vi "lecroy_enable.vi"(0 "VISA in":refnum<visa-resource-name>, 1 "Enable":bool, 2 "Crate":i32, 3 "Card":dbl, 4 "Channel":dbl, 5 "error in":errorcluster, 7 "Num Channels":i32=1) -> (14 "VISA out":refnum<visa-resource-name>, 16 "Read Channel Voltage":dbl, 19 "error out":errorcluster)   [LabVIEW 2018]
uses:
  General_lecroy_command.ctl
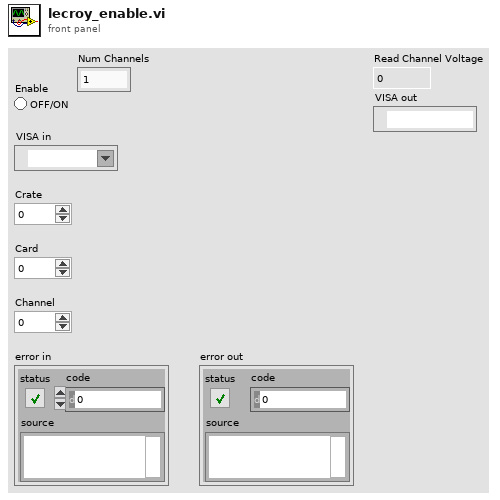
[diagram p1: front panel]
types:
  T1 = enum16{"Monitor", "Demand", "Backup", "All", "None"}
  T2 = typedef "General_lecroy_command.ctl" = string
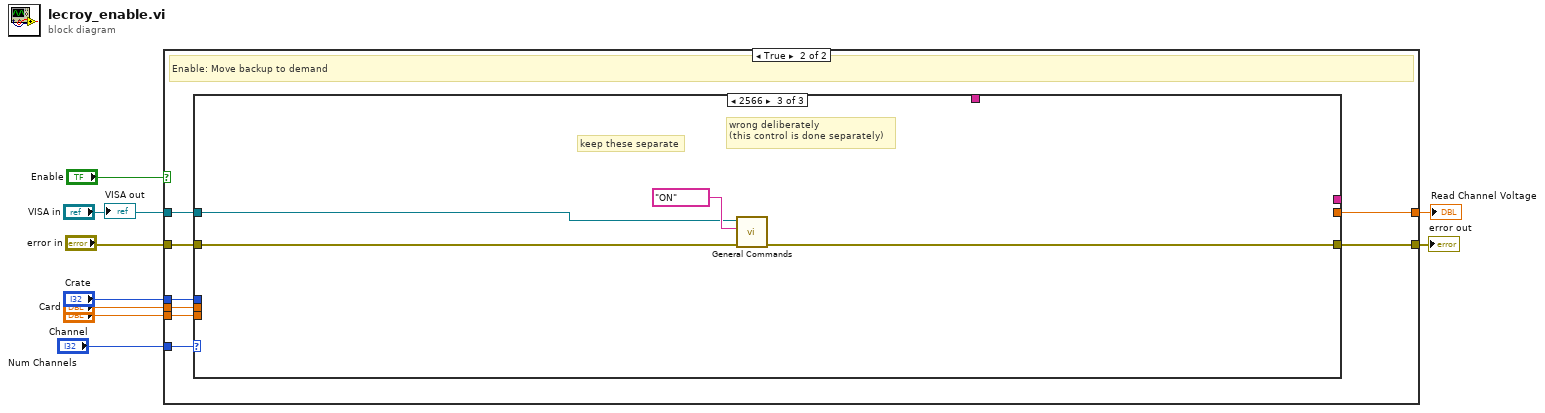
[diagram p0: block diagram]
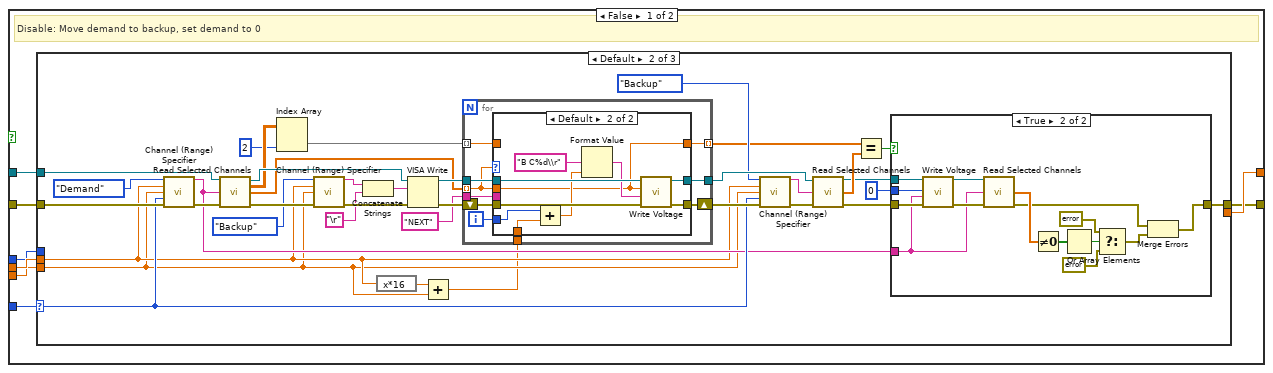
[diagram p2: hidden frame]
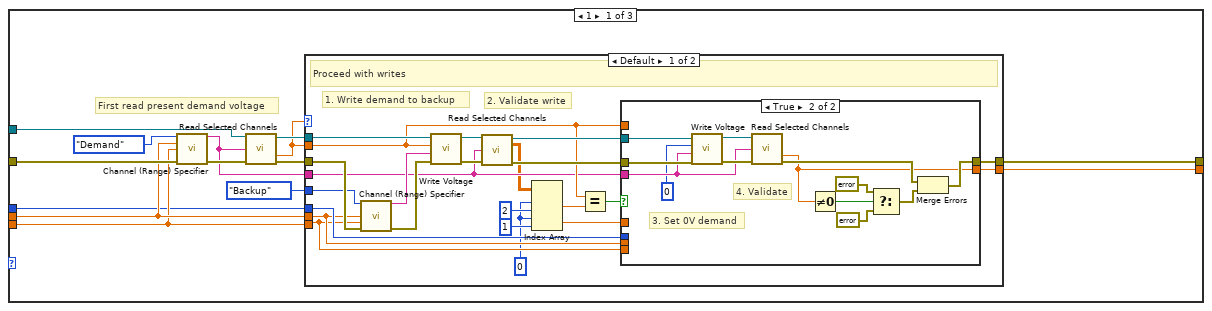
[diagram p3: hidden frame]
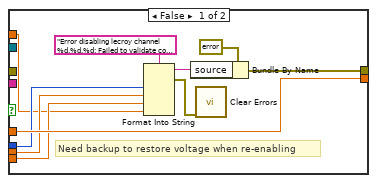
[diagram p4: hidden frame]
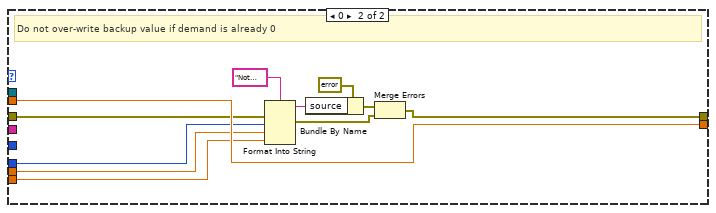
[diagram p5: hidden frame]
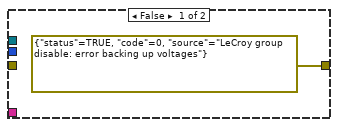
[diagram p6: hidden frame]
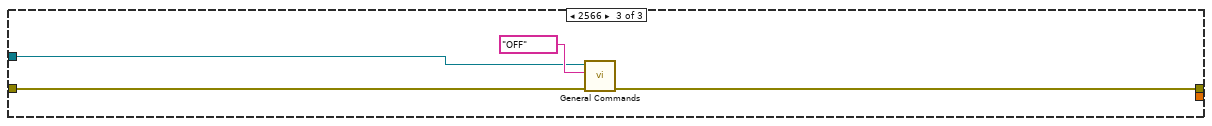
[diagram p8: hidden frame]
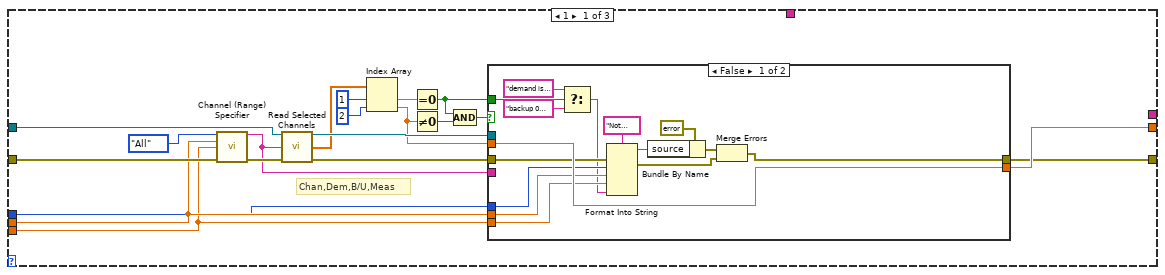
[diagram p9: hidden frame]
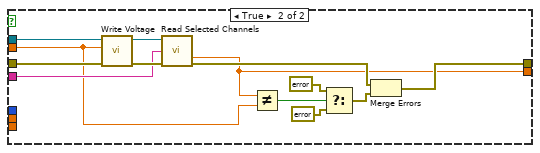
[diagram p10: hidden frame]
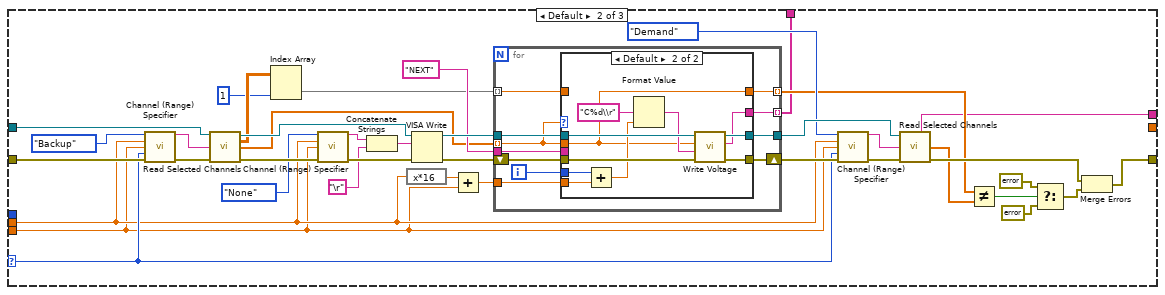
[diagram p11: hidden frame]
diagram:
  n1 = case shown="True" "Enable" {
    tunnel: [w11 w168] -> w2
    tunnel: [w12 w169] -> w3
    tunnel: "error in" -> [w16 w173]
    tunnel: "Channel" -> [w14 w171]
    tunnel: "Card" -> [w15 w172]
    tunnel: "VISA in" -> [w17 w174]
    tunnel: "Crate" -> [w13 w170]
    tunnel: "Num Channels" -> [w10 w167]
    frame False {
      # "Disable: Move demand to backup, set demand to 0"
      n2 = case shown="Default" w10 {
        selector: w10 -> [_ w104 _]
        tunnel: w17 -> [w30 w106 w165]
        tunnel: w16 -> [w29 w105 w164]
        tunnel: w15 -> [w25 w91 _]
        tunnel: w14 -> [w24 w90 _]
        tunnel: w13 -> [w23 _ _]
        tunnel: [w22 _ _] -> w12
        tunnel: [w21 w103 w163] -> w11
        frame 1 {
          # "First read present demand voltage"
          n3 = call "Channel (Range) Specifier.vi"("Buffer"=T1."Demand", "Card"=w25, "Channel"=w24, "error in"=w29) -> ("Channel (Range)"=w26:string, "error out"=w31:errorcluster)  [unwired: 10 in]
          n4 = call "Read Selected Channels.vi"("VISA in"=w30, "C##,##DO###"=w26, "error in"=w31) -> ("VISA out"=w28:refnum<visa-resource-name>, "First Value"=w18:dbl, "error out"=w27:errorcluster)  [unwired: 6 in, 4 out]
          n5 = case shown="Default" w18 {
            tunnel: [w54 w84] -> w22
            tunnel: [w53 w86] -> w21
            tunnel: w18 -> [w38 w84]
            tunnel: w28 -> [w52 _]
            tunnel: w27 -> [w51 w79]
            tunnel: w26 -> [w36 _]
            tunnel: w25 -> [w40 w81]
            tunnel: w24 -> [w39 w82]
            tunnel: w23 -> [w41 w80]
            tunnel: T1."Backup" ("Buffer") -> [w42 _]
            frame Default {
              w32 = 0 ("disabled index (col)")
              # "2. Validate write"
              # "1. Write demand to backup"
              # "Proceed with writes"
              n6 = call "Channel (Range) Specifier.vi"("Buffer"=w42, "Channel"=w40, "Num Channels"=w39, "error in"=w51) -> ("Channel (Range)"=w37:string, "error out"=w50:errorcluster)  [unwired: 10 in]
              n7 = call "Write Voltage.vi"("error in"=w50, "Channel+Range"=w37, "Voltage input"=w38, "VISA in"=w52) -> ("error out"=w49:errorcluster, "VISA out"=w48:refnum<visa-resource-name>)  [unwired: 5 in, 1 out]
              n8 = call "Read Selected Channels.vi"("VISA in"=w48, "C##,##DO###"=w36, "error in"=w49) -> ("VISA out"=w46:refnum<visa-resource-name>, "Channel Array"=w35:dbl[][], "error out"=w47:errorcluster)  [unwired: 6 in, 4 out]
              n9 = Index Array(array=w35, index (row) #1=w32, index (col) #1=2 ("disabled index (col)"), index (row) #2=w32, index (col) #2=1 ("disabled index (col)")) -> (element #1=w44:dbl, element #2=w43:dbl)
              n10 = Equal?(x=w38, y=w44) -> (x = y?=w45:bool)
              n11 = case shown="True" w45 {
                tunnel: [w64 w65] -> w54
                tunnel: [w61 w66] -> w53
                tunnel: w36 -> [_ w73]
                tunnel: w47 -> [_ w77]
                tunnel: w46 -> [_ w76]
                tunnel: w43 -> [w64 _]
                tunnel: w41 -> [w59 _]
                tunnel: w40 -> [w58 _]
                tunnel: w39 -> [w57 _]
                tunnel: w38 -> [w56 _]
                frame False {
                  # "Need backup to restore voltage when re-enabling"
                  n12 = Format Into String(format string="Error disabling lecroy channel %d.%d.%d: Failed to validate copy of demand voltage %d to backup" ("source"), w59, w58, w57, w56) -> (resulting string=w62:string, error out=w55:errorcluster)  [unwired: 2 in]
                  n13 = Bundle By Name(cluster=errorcluster {"status"=TRUE, "code"=0, "source"=""} ("error out"), "source"=w62) -> (w61:errorcluster)
                  n14 = call <vilib>:"Clear Errors.vi"("error in (no error)"=w55) -> ()  [unwired: 5 in, 2 out]
                }
                frame True {
                  # "3. Set 0V demand"
                  # "4. Validate"
                  n15 = call "Write Voltage.vi"("error in"=w77, "Channel+Range"=w73, "Voltage input"=0, "VISA in"=w76) -> ("error out"=w75:errorcluster, "VISA out"=w74:refnum<visa-resource-name>)  [unwired: 5 in, 1 out]
                  n16 = call "Read Selected Channels.vi"("VISA in"=w74, "C##,##DO###"=w73, "error in"=w75) -> ("First Value"=w65:dbl, "error out"=w67:errorcluster)  [unwired: 6 in, 5 out]
                  n17 = Not Equal To 0?(x=w65) -> (x != 0?=w69:bool)
                  n18 = Select(t=errorcluster {"status"=TRUE, "code"=0, "source"="LeCroy disable validation error"} ("error out"), s=w69, f=errorcluster {"status"=FALSE, "code"=0, "source"=""} ("error out")) -> (s? t:f=w68:errorcluster)
                  n19 = Merge Errors(w67, w68) -> (w66:errorcluster)
                }
              }
            }
            frame 0 {
              # "Do not over-write backup value if demand is already 0"
              n20 = Format Into String(format string="Not enabling channel %d.%d.%d:\ndemand is 0 (channel already disabled)" ("source"), error in=w79, w80, w81, w82) -> (resulting string=w87:string, error out=w83:errorcluster)  [unwired: 1 in]
              n21 = Bundle By Name(cluster=errorcluster {"status"=TRUE, "code"=0, "source"=""} ("error out"), "source"=w87) -> (w85:errorcluster)
              n22 = Merge Errors(w85, w83) -> (w86:errorcluster)
            }
          }
        }
        frame Default {
          n23 = call "Channel (Range) Specifier.vi"("Buffer"=T1."Demand", "Card"=w91, "Channel"=w90, "Num Channels"=w104, "error in"=w105) -> ("Channel (Range)"=w93:string, "error out"=w124:errorcluster)  [unwired: 9 in]
          n24 = call "Read Selected Channels.vi"("VISA in"=w106, "C##,##DO###"=w93, "error in"=w124) -> ("VISA out"=w120:refnum<visa-resource-name>, "Channel Array"=w98:dbl[][], "Selected Buffer"=w101:dbl[], "error out"=w122:errorcluster)  [unwired: 6 in, 3 out]
          n25 = Index Array(array=w98, index (col)=2 ("disabled index (col)")) -> (element=w96:dbl[])  [unwired: 1 in]
          n26 = call "Channel (Range) Specifier.vi"("Buffer"=T1."Backup", "Card"=w91, "Channel"=w90, "error in"=w122) -> ("Channel (Range)"=w118:string, "error out"=w116:errorcluster)  [unwired: 10 in]
          n27 = Concatenate Strings(w118, "\r") -> (w117:string)
          n28 = expression code="x*16"(w91) -> (w92:dbl)
          n29 = VISA Write(VISA resource name=w120, write buffer=w117, error in (no error)=w116) -> (VISA resource name out=w119:refnum<visa-resource-name>, error out=w121:errorcluster)  [unwired: 1 out]
          n30 = Add(x=w92, y=w90) -> (x+y=w89:dbl)
          n31 = for {
            shift-right: [w149] -> w115
            shift-left: w121 -> [w147]
            tunnel: w119 -> [w146]
            tunnel: [w148] -> w113
            tunnel: w101 -> [w143] mode=indexing
            tunnel: "NEXT" ("Channel (Range)") -> [w145]
            tunnel: [w144] -> w99 mode=indexing
            tunnel: w96 -> [w142] mode=indexing
            tunnel: w89 -> [w140]
            i -> [w141]
            n32 = case shown="Default" w143 {
              tunnel: [w151 w162] -> w149
              tunnel: [w150 w161] -> w148
              tunnel: w147 -> [w151 w160]
              tunnel: w146 -> [w150 w159]
              tunnel: w143 -> [_ w153]
              tunnel: w145 -> [_ _]
              tunnel: [w152 w153] -> w144
              tunnel: w142 -> [w152 _]
              tunnel: w141 -> [_ w158]
              tunnel: w140 -> [_ w157]
              frame 0 {
              }
              frame Default {
                n33 = Add(x=w158, y=w157) -> (x+y=w155:dbl)
                n34 = Format Value(format string="B C%d\\r" ("Channel (Range)"), value (0)=w155) -> (output string=w154:string)  [unwired: 1 in]
                n35 = call "Write Voltage.vi"("error in"=w160, "Channel+Range"=w154, "Voltage input"=w153, "VISA in"=w159) -> ("error out"=w162:errorcluster, "VISA out"=w161:refnum<visa-resource-name>)  [unwired: 5 in, 1 out]
              }
            }
          }
          n36 = call "Channel (Range) Specifier.vi"("Buffer"=T1."Backup", "Card"=w91, "Channel"=w90, "Num Channels"=w104, "error in"=w115) -> ("Channel (Range)"=w112:string, "error out"=w114:errorcluster)  [unwired: 9 in]
          n37 = call "Read Selected Channels.vi"("VISA in"=w113, "C##,##DO###"=w112, "error in"=w114) -> ("VISA out"=w95:refnum<visa-resource-name>, "Selected Buffer"=w102:dbl[], "error out"=w123:errorcluster)  [unwired: 6 in, 4 out]
          n38 = Equal?(x=w99, y=w102) -> (x = y?=w100:bool)
          n39 = case shown="True" w100 {
            tunnel: w123 -> [_ w133]
            tunnel: [errorcluster {"status"=TRUE, "code"=0, "source"="LeCroy group disable: error backing up voltages"} ("error out") w136] -> w103
            tunnel: w95 -> [_ w132]
            tunnel: 0 ("Voltage input") -> [_ w131]
            tunnel: w93 -> [_ w128]
            frame False {
            }
            frame True {
              n40 = call "Write Voltage.vi"("error in"=w133, "Channel+Range"=w128, "Voltage input"=w131, "VISA in"=w132) -> ("error out"=w130:errorcluster, "VISA out"=w129:refnum<visa-resource-name>)  [unwired: 5 in, 1 out]
              n41 = call "Read Selected Channels.vi"("VISA in"=w129, "C##,##DO###"=w128, "error in"=w130) -> ("Selected Buffer"=w127:dbl[], "error out"=w126:errorcluster)  [unwired: 6 in, 5 out]
              n42 = Not Equal To 0?(x=w127) -> (x != 0?=w135:bool[])
              n43 = Or Array Elements(Boolean array=w135) -> (logical OR=w134:bool)
              n44 = Select(t=errorcluster {"status"=TRUE, "code"=0, "source"="LeCroy group enable validation error"} ("error out"), s=w134, f=errorcluster {"status"=FALSE, "code"=0, "source"=""} ("error out")) -> (s? t:f=w139:errorcluster)
              n45 = Merge Errors(w126, w139) -> (w136:errorcluster)
            }
          }
        }
        frame 2566 {
          n46 = call "General Commands.vi"("error in"=w164, "Action"=T2 "OFF", "VISA in"=w165) -> ("error out"=w163:errorcluster)  [unwired: 6 in, 2 out]
        }
      }
    }
    frame True {
      # "Enable: Move backup to demand"
      n47 = case shown="2566" w167 {
        selector: w167 -> [_ w234 _]
        tunnel: w174 -> [w193 w260 w288]
        tunnel: w173 -> [w192 w259 w287]
        tunnel: w172 -> [w184 w227 _]
        tunnel: w171 -> [w183 w226 _]
        tunnel: w170 -> [w182 _ _]
        tunnel: [w181 _ _] -> w169
        tunnel: [w180 w257 w289] -> w168
        tunnel: [_ w225 _] -> _
        tunnel: [_ w223 _] -> _
        frame 1 {
          # "Chan,Dem,B/U,Meas"
          n48 = call "Channel (Range) Specifier.vi"("Buffer"=T1."All", "Card"=w184, "Channel"=w183, "error in"=w192) -> ("Channel (Range)"=w189:string, "error out"=w194:errorcluster)  [unwired: 10 in]
          n49 = call "Read Selected Channels.vi"("VISA in"=w193, "C##,##DO###"=w189, "error in"=w194) -> ("VISA out"=w191:refnum<visa-resource-name>, "Selected Buffer"=w178:dbl[], "error out"=w190:errorcluster)  [unwired: 6 in, 4 out]
          n50 = Index Array(array=w178, index #1=1 ("disabled index (col)"), index #2=2 ("disabled index (col)")) -> (element #1=w188:dbl, element #2=w185:dbl)
          n51 = Equal To 0?(x=w188) -> (x = 0?=w175:bool)
          n52 = Not Equal To 0?(x=w185) -> (x != 0?=w187:bool)
          n53 = Compound Arithmetic op=AND(w175, w187) -> (w186:bool)
          n54 = case shown="False" w186 {
            tunnel: [w203 w210] -> w181
            tunnel: [w205 w211] -> w180
            tunnel: w185 -> [w203 w213]
            tunnel: w191 -> [_ w220]
            tunnel: w190 -> [w197 w219]
            tunnel: w189 -> [_ w218]
            tunnel: w184 -> [w199 _]
            tunnel: w183 -> [w200 _]
            tunnel: w182 -> [w198 _]
            tunnel: w175 -> [w195 _]
            frame False {
              n55 = Select(t="demand is not 0 (channel already enabled)" ("source"), s=w195, f="backup 0 (channel has no Vset)" ("source")) -> (s? t:f=w196:string)
              n56 = Format Into String(format string="Not enabling channel %d.%d.%d: %s" ("source"), error in=w197, w198, w199, w200, w196) -> (resulting string=w206:string, error out=w201:errorcluster)  [unwired: 1 in]
              n57 = Bundle By Name(cluster=errorcluster {"status"=TRUE, "code"=0, "source"=""} ("error out"), "source"=w206) -> (w204:errorcluster)
              n58 = Merge Errors(w204, w201) -> (w205:errorcluster)
            }
            frame True {
              n59 = call "Write Voltage.vi"("error in"=w219, "Voltage input"=w213, "VISA in"=w220) -> ("error out"=w222:errorcluster, "VISA out"=w221:refnum<visa-resource-name>)  [unwired: 6 in, 1 out]
              n60 = call "Read Selected Channels.vi"("VISA in"=w221, "C##,##DO###"=w218, "error in"=w222) -> ("First Value"=w210:dbl, "error out"=w212:errorcluster)  [unwired: 6 in, 5 out]
              n61 = Not Equal?(x=w210, y=w213) -> (x != y?=w215:bool)
              n62 = Select(t=errorcluster {"status"=TRUE, "code"=0, "source"="LeCroy enable validation error"} ("error out"), s=w215, f=errorcluster {"status"=FALSE, "code"=0, "source"=""} ("error out")) -> (s? t:f=w214:errorcluster)
              n63 = Merge Errors(w212, w214) -> (w211:errorcluster)
            }
          }
        }
        frame Default {
          n64 = call "Channel (Range) Specifier.vi"("Buffer"=T1."Backup", "Card"=w227, "Channel"=w226, "Num Channels"=w234, "error in"=w259) -> ("Channel (Range)"=w258:string, "error out"=w261:errorcluster)  [unwired: 9 in]
          n65 = call "Read Selected Channels.vi"("VISA in"=w260, "C##,##DO###"=w258, "error in"=w261) -> ("VISA out"=w247:refnum<visa-resource-name>, "Channel Array"=w232:dbl[][], "Selected Buffer"=w240:dbl[], "error out"=w250:errorcluster)  [unwired: 6 in, 3 out]
          n66 = Index Array(array=w232, index (col)=1 ("disabled index (col)")) -> (element=w230:dbl[])  [unwired: 1 in]
          n67 = call "Channel (Range) Specifier.vi"("Buffer"=T1."None", "Card"=w227, "Channel"=w226, "error in"=w250) -> ("Channel (Range)"=w245:string, "error out"=w243:errorcluster)  [unwired: 10 in]
          n68 = Concatenate Strings(w245, "\r") -> (w244:string)
          n69 = expression code="x*16"(w227) -> (w228:dbl)
          n70 = VISA Write(VISA resource name=w247, write buffer=w244, error in (no error)=w243) -> (VISA resource name out=w246:refnum<visa-resource-name>, error out=w248:errorcluster)  [unwired: 1 out]
          n71 = Add(x=w228, y=w226) -> (x+y=w224:dbl)
          n72 = for {
            shift-right: [w272] -> w238
            shift-left: w248 -> [w270]
            tunnel: w246 -> [w269]
            tunnel: [w271] -> w236
            tunnel: w240 -> [w267] mode=indexing
            tunnel: "NEXT" ("Channel (Range)") -> [w268]
            tunnel: w230 -> [w266] mode=indexing
            tunnel: [w265] -> w229 mode=indexing
            tunnel: w224 -> [w264]
            tunnel: [w262] -> w223 mode=indexing
            i -> [w263]
            n73 = case shown="Default" w267 {
              tunnel: [w273 w286] -> w272
              tunnel: [w274 w285] -> w271
              tunnel: w270 -> [w273 w284]
              tunnel: w269 -> [w274 w283]
              tunnel: w267 -> [_ w277]
              tunnel: w268 -> [_ _]
              tunnel: w266 -> [w275 _]
              tunnel: [w275 w277] -> w265
              tunnel: w264 -> [_ w281]
              tunnel: w263 -> [_ w280]
              tunnel: [_ w276] -> w262
              frame 0 {
              }
              frame Default {
                n74 = Add(x=w280, y=w281) -> (x+y=w279:dbl)
                n75 = Format Value(format string="C%d\\r" ("Channel (Range)"), value (0)=w279) -> (output string=w278:string)  [unwired: 1 in]
                n76 = call "Write Voltage.vi"("error in"=w284, "Channel+Range"=w278, "Voltage input"=w277, "VISA in"=w283) -> ("error out"=w286:errorcluster, "read buffer"=w276:string, "VISA out"=w285:refnum<visa-resource-name>)  [unwired: 5 in]
              }
            }
          }
          n77 = call "Channel (Range) Specifier.vi"("Buffer"=T1."Demand", "Card"=w227, "Channel"=w226, "Num Channels"=w234, "error in"=w238) -> ("Channel (Range)"=w235:string, "error out"=w237:errorcluster)  [unwired: 9 in]
          n78 = call "Read Selected Channels.vi"("VISA in"=w236, "C##,##DO###"=w235, "error in"=w237) -> ("Final Output"=w225:string, "Selected Buffer"=w239:dbl[], "error out"=w251:errorcluster)  [unwired: 6 in, 4 out]
          n79 = Not Equal?(x=w229, y=w239) -> (x != y?=w253:bool)
          n80 = Select(t=errorcluster {"status"=TRUE, "code"=0, "source"="LeCroy group enable validation error"} ("error out"), s=w253, f=errorcluster {"status"=FALSE, "code"=0, "source"=""} ("error out")) -> (s? t:f=w252:errorcluster)
          n81 = Merge Errors(w251, w252) -> (w257:errorcluster)
        }
        frame 2566 {
          # "wrong deliberately\n(this control is done separately)"
          # "keep these separate"
          n82 = call "General Commands.vi"("error in"=w287, "Action"=T2 "ON", "VISA in"=w288) -> ("error out"=w289:errorcluster)  [unwired: 6 in, 2 out]
        }
      }
    }
  }
  "error out" <- w2
  "Read Channel Voltage" <- w3
  "VISA out" <- "VISA in"
